vi "R1C_GPIO_A.vi"(0 "rsv":u32, 3 "op_red_led":u32, 4 "io_red_led":u32, 5 "op_green_led":u32, 6 "tx_io_sw1":u32, 7 "pd_rxcomb_other":u32, 8 "tx_io_sw2":u32, 11 "pd_rxif12_txif2":u32) -> (2 "GPIO_A":u32)   [LabVIEW 2018]
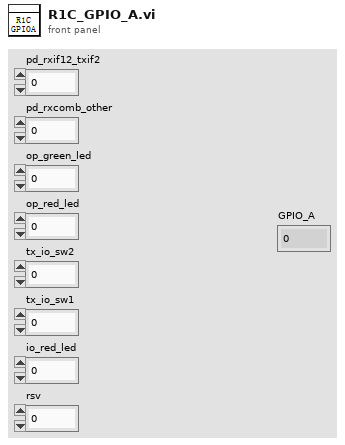
[diagram p1: front panel]
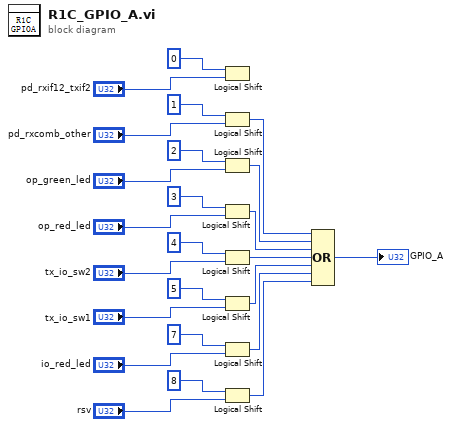
[diagram p0: block diagram]
diagram:
  n1 = Logical Shift(y=i16 0, x="pd_rxif12_txif2") -> ()  [unwired: 1 out]
  n2 = Logical Shift(y=i16 1, x="pd_rxcomb_other") -> (x << y=w8:u32)
  n3 = Logical Shift(y=i16 2, x="op_green_led") -> (x << y=w7:u32)
  n4 = Logical Shift(y=i16 3, x="op_red_led") -> (x << y=w6:u32)
  n5 = Logical Shift(y=i16 4, x="tx_io_sw2") -> (x << y=w5:u32)
  n6 = Logical Shift(y=i16 5, x="tx_io_sw1") -> (x << y=w4:u32)
  n7 = Logical Shift(y=i16 7, x="io_red_led") -> (x << y=w3:u32)
  n8 = Logical Shift(y=i16 8, x="rsv") -> (x << y=w2:u32)
  n9 = Compound Arithmetic op=OR(w8, w7, w6, w5, w4, w3, w2) -> (→"GPIO_A":u32)
